vi "Test_MergeErrorsPublication_ErrorCluster_ErrorMerged.vi"(8 "error in (no error)":errorcluster, 11 "TestCase in":refnum<class "TestPublicationPolicy.lvclass">) -> (0 "error out":errorcluster, 3 "TestCase out":refnum<class "TestPublicationPolicy.lvclass">)   [LabVIEW 2017, in "TestPublicationPolicy.lvclass"]
uses:
  TestPublicationPolicy.lvclass
  gpm_packages/@cs/mva-core/Source/IMediator/MutexedPublishRequest/MutexedPublishRequest.lvclass
  gpm_packages/@cs/mva-core/Source/IMediator/IPublicationPolicy/IPublicationPolicy.lvclass
  gpm_packages/@cs/mva-core/Source/PublicationPolicy/MergeErrorsPublication/MergeErrorsPublication.lvclass
  gpm_packages/@cs/transport/Source/Concrete/NotifierTransport/NotifierTransport.lvclass
  C:/Git/mva-framework/Source/Framework/IMediator/IPublicationPolicy/IPublicationPolicy.lvclass
  C:/Git/mva-framework/gpm_packages/@cs/transport/Source/ITransport/ITransport.lvclass
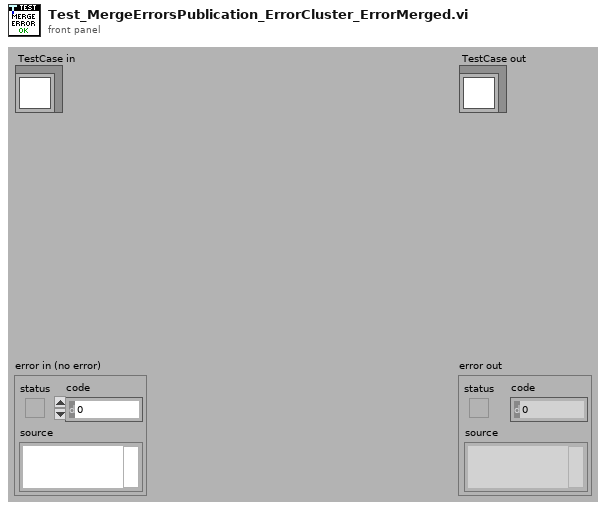
[diagram p1: front panel]
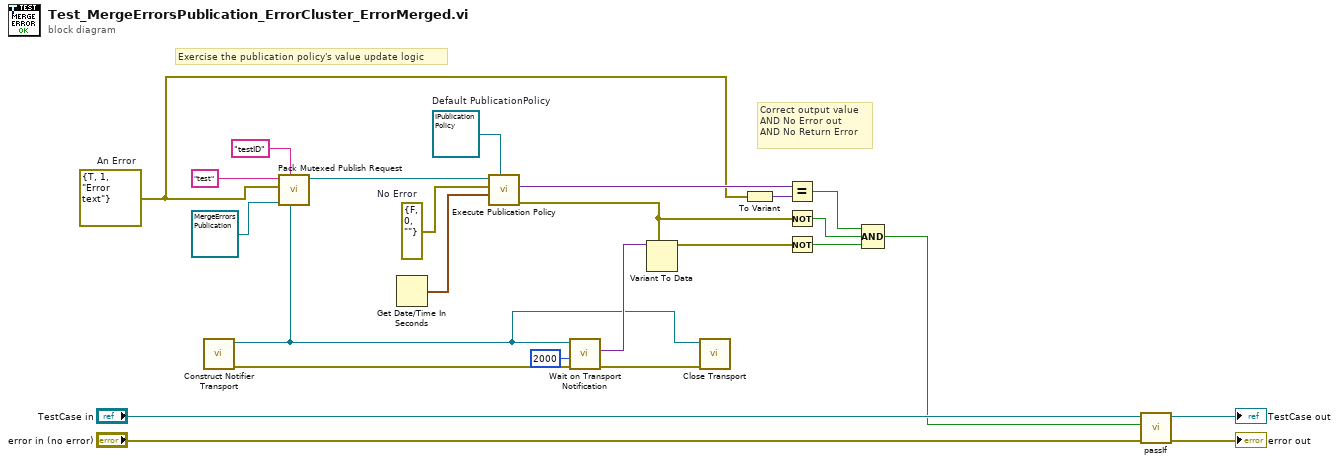
[diagram p0: block diagram]
diagram:
  w4 = errorcluster {"status"=TRUE, "code"=1, "source"="Error text"}  # An Error
  w17 = refnum<class "IPublicationPolicy.lvclass"> refnum  # Default PublicationPolicy
  w21 = errorcluster {"status"=FALSE, "code"=0, "source"=""}  # No Error
  # "Correct output value\nAND No Error out\nAND No Return Error"
  # "Exercise the publication policy's value update logic"
  n1 = call "Construct Notifier Transport.vi"() -> ("error out"=w14:errorcluster, "NotifierTransport"=w2:refnum<class "NotifierTransport.lvclass">)  [unwired: 10 in]
  n2 = call "Pack Mutexed Publish Request.vi"("Return Error Transport"=w2, "Publisher ID"="testID", "error in (no error)"=refnum<class "MergeErrorsPublication.lvclass"> refnum ("PublicationPolicy.lvlib:MergeErrorsPublication.lvclass"), "Datum Value or Type"=w4, "Datum Name"="test") -> ("MutexedPublishRequest Out"=w19:refnum<class "MutexedPublishRequest.lvclass">)  [unwired: 5 in, 1 out]
  n3 = Get Date/Time In Seconds() -> (seconds since 1Jan1904=w20:timestamp)
  n4 = call-dynamic "Execute Publication Policy.vi"("Default PublicationPolicy"=w17, "Last Publish Time"=w20, "Last Published Value"=w21, "MutexedPublishRequest"=w19) -> ("error out (Reject Publication)"=w6:errorcluster, "Value to Publish"=w11:variant)  [unwired: 5 in, 1 out]
  n5 = call "Wait on Transport Notification.vi"("error in (no error)"=w14, "Timeout In ms (-1)"=2000, "NotifierTransport"=w2) -> ("error out"=w1:errorcluster, "Data"=w12:variant)  [unwired: 6 in, 1 out]
  n6 = Variant To Data(type=w6, Variant=w12) -> (data=w9:errorcluster)  [unwired: 1 in, 1 out]
  n7 = call-dynamic "Close Transport.vi"("error in (no error)"=w1, "NotifierTransport"=w2) -> ()  [unwired: 9 in, 1 out]
  n8 = To Variant(anything=w4) -> (Variant=w10:variant)
  n9 = Equal?(x=w11, y=w10) -> (x = y?=w8:bool)
  n10 = Not(x=w6) -> (.not. x?=w5:bool)
  n11 = Not(x=w9) -> (.not. x?=w7:bool)
  n12 = Compound Arithmetic op=AND(w8, w5, w7) -> (w3:bool)
  n13 = call-dynamic "passIf.vi"("error in (no error)"="error in (no error)", "pass"=w3, "TestCase in"="TestCase in") -> ("error out"=→"error out":errorcluster, "TestCase out"=→"TestCase out":refnum<class "TestPublicationPolicy.lvclass">)  [unwired: 7 in]
